vi "Update Drive Status.vi"(8 "error in (no error)":errorcluster, 10 "Drive Status In":u8, 11 "Data In []":dbl[](array[numeric])) -> (0 "error out":errorcluster, 2 "Drive Status Out":u8, 3 "Data Out []":dbl[](array[numeric]))   [LabVIEW 2016, in "Scan Engine Custom Device.lvlib" / "DS402.lvlib"]
uses:
  DS402.lvlib
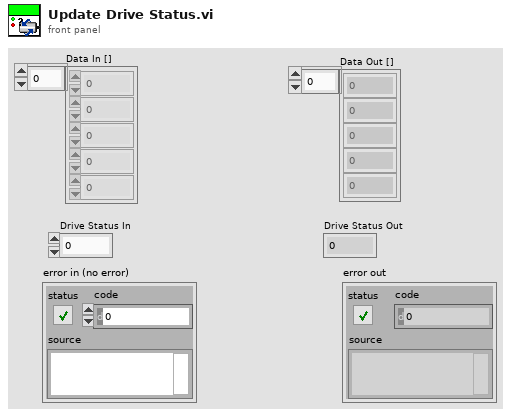
[diagram p1: front panel]
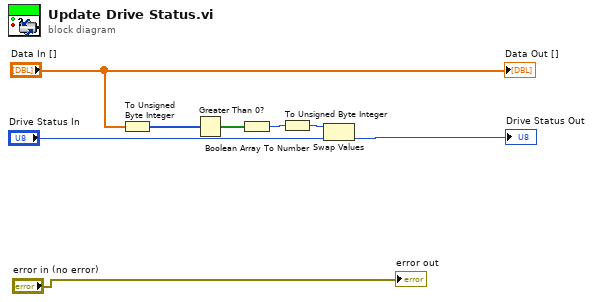
[diagram p0: block diagram]
diagram:
  n1 = To Unsigned Byte Integer(number="Data In []") -> (unsigned 8bit integer=w6:u8[])
  n2 = Greater Than 0?(x=w6) -> (x > 0?=w5:bool[])
  n3 = Boolean Array To Number(Boolean array=w5) -> (number=w4:u32)
  n4 = To Unsigned Byte Integer(number=w4) -> (unsigned 8bit integer=w3:u8)
  n5 = Swap Values(12:w3, 14:"Drive Status In") -> (3:→"Drive Status Out":u8)  [unwired: 1 in, 1 out]
  "Data Out []" <- "Data In []"
  "error out" <- "error in (no error)"
